vi "Motion_Profile_Setup_Send.vi"(7 "name or relative path":string) -> ()   [LabVIEW 2017]
uses:
  <vilib>/Rock Robotics/WPI/ThirdParty/Phoenix-LabVIEW/Motor Controller/Controls/CTRE_Phoenix_MotorControl_TrajectoryPointTimeDur.ctl
  <vilib>/Utility/file.llb/Read Delimited Spreadsheet (DBL).vi
panel:
  out "Total Run TIme":dbl
  out "Done??":bool
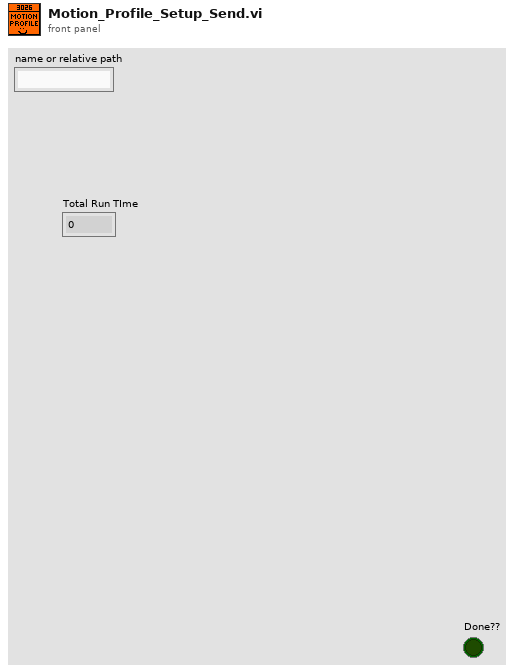
[diagram p1: front panel]
types:
  T1 = typedef "WPI_MotorControlDeviceRef.ctl" = cluster{"DeviceStatus":errorcluster, "Type":T2, "PWM":cluster{"PWM Channel":T3, "DeadBand":T4}, "CAN":cluster{"Device Number":u8, "SetOutput VI Ref":variant, "GetOutput VI Ref":variant, "Enable VI Ref":variant, "Disable VI Ref":variant, "Data":variant}, "Invert":bool, "DIO PWM":cluster{"PWM \"Enable\" Channel":T3, "DIOChannel":T5, "PWM Rate":dbl}}
  T2 = typedef "WPI_MotorControlType.ctl" = enum16{"PWM", "CAN", "DIO PWM"}
  T3 = typedef "FPGA_DIOPWMChannel.ctl" = enum8{"PWM 0", "PWM 1", "PWM 2", "PWM 3", "PWM 4", "PWM 5", "PWM 6", "PWM 7", "PWM 8", "PWM 9", "PWM MXP 0", "PWM MXP 1", "PWM MXP 2", "PWM MXP 3", "PWM MXP 4", "PWM MXP 5", "PWM MXP 6", "PWM MXP 7", "PWM MXP 8", "PWM MXP 9", "Invalid"}
  T4 = typedef "WPI_PWMDeadband.ctl" = cluster{"Name":string, "maxPositivePwm":i32, "minPositivePwm":i32, "centerPwm":i32, "maxNegativePwm":i32, "minNegativePwm":i32, "angularRange":u16}
  T5 = typedef "FPGA_DIOChannel.ctl" = enum8{"DIO 0", "DIO 1", "DIO 2", "DIO 3", "DIO 4", "DIO 5", "DIO 6", "DIO 7", "DIO 8", "DIO 9", "DIO MXP 0", "DIO MXP 1", "DIO MXP 2", "DIO MXP 3", "DIO MXP 4", "DIO MXP 5", "DIO MXP 6", "DIO MXP 7", "DIO MXP 8", "DIO MXP 9", "DIO MXP 10", "DIO MXP 11", "DIO MXP 12", "DIO MXP 13", "DIO MXP 14", "DIO MXP 15", "SPI Port CS1", "SPI Port CS2", "SPI Port CS3", "SPI Port MISO", "SPI Port MOSI", "Invalid"}
  T6 = typedef "CTRE_Phoenix_MotorControl_TrajectoryPointTimeDur.ctl" = i32
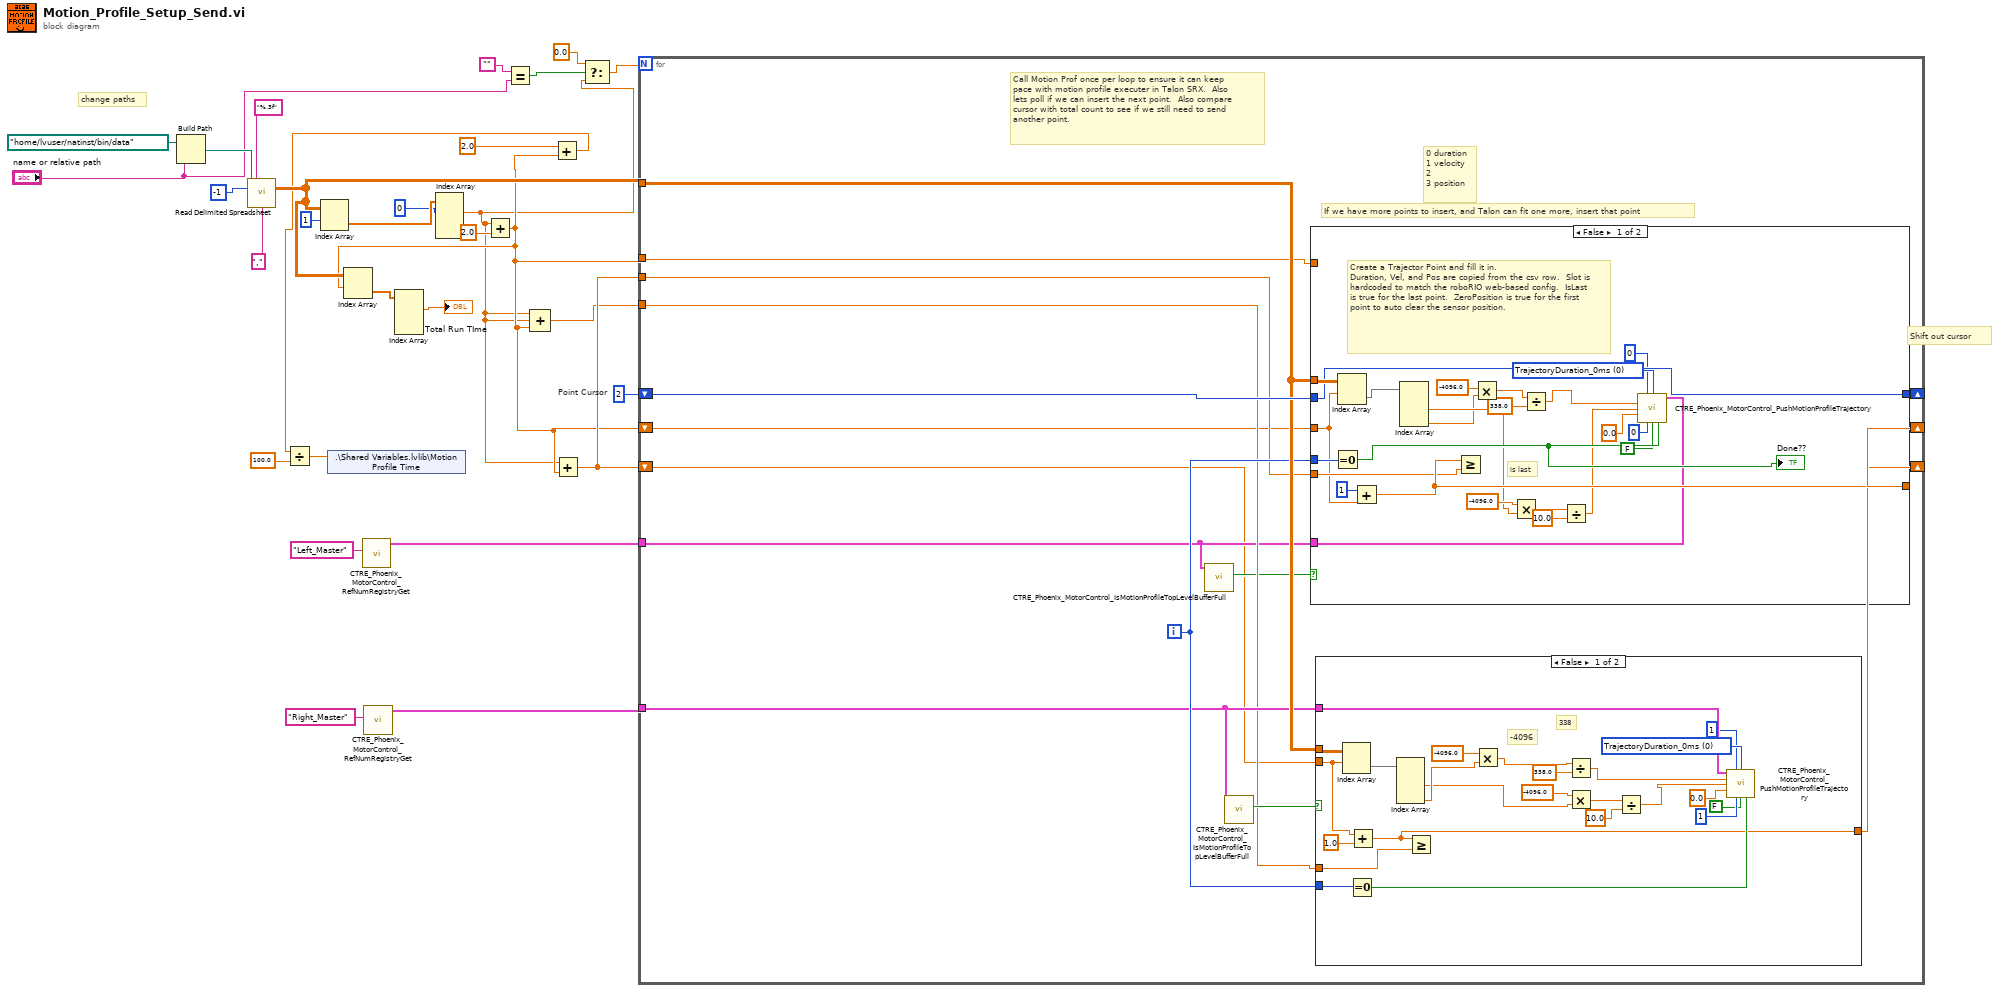
[diagram p0: block diagram]
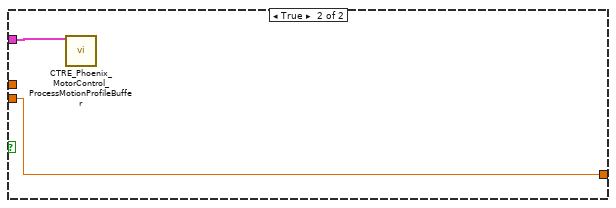
[diagram p2: hidden frame]
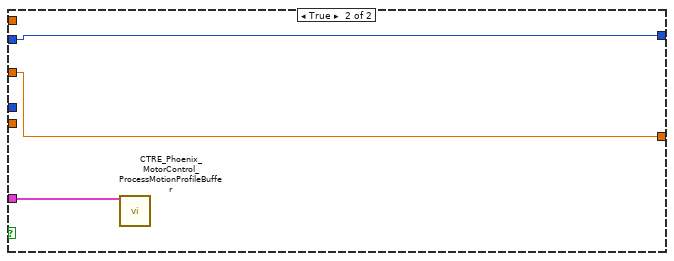
[diagram p3: hidden frame]
diagram:
  w29 = 2  # Point Cursor
  # "change paths"
  # "Shift out cursor"
  n1 = Build Path(base path=path "/home/lvuser/natinst/bin/data", name or relative path="name or relative path") -> (appended path=w28:path)
  n2 = call-poly <vilib>:"Read Delimited Spreadsheet.vi"("file path (dialog if empty)"=w28, "format (%.3f)"="%.3f", "number of rows (all:-1)"=-1, "delimiter (\\t)"="," ("delimiter (\\t)")) -> ("all rows"=w17:dbl[][])  [unwired: 6 in, 5 out]
  n3 = Index Array(array=w17, index (row)=1) -> (element=w25:dbl[])  [unwired: 1 in]
  n4 = call <vilib>:"CTRE_Phoenix_MotorControl_RefNumRegistryGet.vi"("refnum name"="Left_Master") -> ("PhoenixMotorControlDevRef"=w2:T1)  [unwired: 9 in, 1 out]
  n5 = call <vilib>:"CTRE_Phoenix_MotorControl_RefNumRegistryGet.vi"("refnum name"="Right_Master") -> ("PhoenixMotorControlDevRef"=w1:T1)  [unwired: 9 in, 1 out]
  n6 = Index Array(array=w25, index #1=0 ("index")) -> (element #1=w8:dbl)  [unwired: 3 in, 3 out]
  n7 = Add(x=w8, y=2.0) -> (x+y=w15:dbl)
  n8 = Index Array(array=w17, index (row)=w15) -> (element=w16:dbl[])  [unwired: 1 in]
  n9 = Index Array(array=w16) -> (element #1=→"Total Run TIme":dbl)  [unwired: 4 in, 3 out]
  n10 = Equal?(x="", y="name or relative path") -> (x = y?=w4:bool)
  n11 = Compound Arithmetic op=ADD(w8, w8, w15) -> (w18:dbl)
  n12 = Add(x=2.0, y=w15) -> (x+y=w9:dbl)
  n13 = Divide(x=w9, y=100.0) -> (x/y=w11:dbl)
  n14 = shared-variable ".\\Shared Variables.lvlib\\Motion Profile Time"(w11) -> ()  [unwired: 1 in, 1 out]
  n15 = Add(x=w8, y=w15) -> (x+y=w19:dbl)
  n16 = Select(t=0.0, s=w4, f=w8) -> (s? t:f=w7:dbl)
  n17 = for {
    N: w7 -> [_]
    tunnel: w17 -> [w44]
    shift-right: [w33] -> _
    shift-left: w29 -> [w45]
    tunnel: w15 -> [w40]
    tunnel: w2 -> [w37]
    tunnel: w1 -> [w41]
    tunnel: w19 -> [w39]
    tunnel: w18 -> [w38]
    shift-right: [w34] -> _
    shift-left: w19 -> [w31]
    shift-right: [w35] -> _
    shift-left: w15 -> [w32]
    i -> [w43]
    # "0 duration\n1 velocity \n2 \n3 position"
    # "If we have more points to insert, and Talon can fit one more, insert that point"
    # "Call Motion Prof once per loop to ensure it can keep pace with motion profile executer in Talon SRX.  Also lets poll if we can insert the next point.  Also compare cursor with total count to see if we still need to send another point."
    n18 = call <vilib>:"CTRE_Phoenix_MotorControl_IsMotionProfileTopLevelBufferFull.vi"("PhoenixMotorControlDevRef"=w37) -> ("Is Motion Profile Top Level Buffer Full?"=w36:bool)  [unwired: 8 in, 2 out]
    n19 = call <vilib>:"CTRE_Phoenix_MotorControl_IsMotionProfileTopLevelBufferFull.vi"("PhoenixMotorControlDevRef"=w41) -> ("Is Motion Profile Top Level Buffer Full?"=w42:bool)  [unwired: 8 in, 2 out]
    n20 = case shown="False" w36 {
      tunnel: w44 -> [w96 _]
      tunnel: [w93 w99] -> w35
      tunnel: w45 -> [w86 w98]
      tunnel: w37 -> [w87 w97]
      tunnel: w43 -> [w92 _]
      tunnel: w40 -> [_ _]
      tunnel: w39 -> [w88 _]
      tunnel: w32 -> [w75 w99]
      tunnel: [w86 w98] -> w33
      frame False {
        w85 = T6 0 items=["TrajectoryDuration_0ms"=0, "TrajectoryDuration_5ms"=5, "TrajectoryDuration_10ms"=10, "TrajectoryDuration_20ms"=20, "TrajectoryDuration_30ms"=30, "TrajectoryDuration_40ms"=40, "TrajectoryDuration_50ms"=50, "TrajectoryDuration_100ms"=100] ("durationMs")
        # "is last"
        # "Create a Trajector Point and fill it in.\nDuration, Vel, and Pos are copied from the csv row.  Slot is hardcoded to match the roboRIO web-based config.  IsLast is true for the last point.  ZeroPosition is true for the first point to auto clear the sensor position."
        n21 = Equal To 0?(x=w92) -> (x = 0?=w91:bool)
        "Done??" <- w91
        n22 = Index Array(array=w96, index (row)=w75) -> (element=w94:dbl[])  [unwired: 1 in]
        n23 = Add(x=u32 1, y=w75) -> (x+y=w93:dbl)
        n24 = Index Array(array=w94) -> (element #2=w78:dbl, element #4=w77:dbl)  [unwired: 4 in, 2 out]
        n25 = Greater Or Equal?(x=w93, y=w88) -> ()  [unwired: 1 out]
        n26 = Multiply(x=-4096.0, y=w77) -> (x*y=w73:dbl)
        n27 = Multiply(x=-4096.0, y=w78) -> (x*y=w80:dbl)
        n28 = Divide(x=w73, y=338.0) -> (x/y=w72:dbl)
        n29 = Divide(x=w80, y=10.0) -> (x/y=w76:dbl)
        n30 = call <vilib>:"CTRE_Phoenix_MotorControl_PushMotionProfileTrajectory.vi"("PhoenixMotorControlDevRef"=w87, "profileSlotSelect1"=0, "durationMs"=w85, "position"=w72, "velocity"=w76, "headingDeg"=0.0, "profileSlotSelect0"=0 ("profileSlotSelect"), "isLastPoint?"=FALSE, "Zero Position?"=w91) -> ()  [unwired: 5 in, 2 out]
      }
      frame True {
        n31 = call <vilib>:"CTRE_Phoenix_MotorControl_ProcessMotionProfileBuffer.vi"("PhoenixMotorControlDevRef"=w97) -> ()  [unwired: 13 in, 2 out]
      }
    }
    n32 = case shown="False" w42 {
      tunnel: w41 -> [w62 w70]
      tunnel: w44 -> [w69 _]
      tunnel: w43 -> [w67 _]
      tunnel: w38 -> [w61 _]
      tunnel: w31 -> [w49 w71]
      tunnel: [w60 w71] -> w34
      frame False {
        w59 = T6 0 items=["TrajectoryDuration_0ms"=0, "TrajectoryDuration_5ms"=5, "TrajectoryDuration_10ms"=10, "TrajectoryDuration_20ms"=20, "TrajectoryDuration_30ms"=30, "TrajectoryDuration_40ms"=40, "TrajectoryDuration_50ms"=50, "TrajectoryDuration_100ms"=100] ("durationMs")
        # "338"
        # "-4096"
        n33 = Index Array(array=w69, index (row)=w49) -> (element=w68:dbl[])  [unwired: 1 in]
        n34 = Equal To 0?(x=w67) -> (x = 0?=w63:bool)
        n35 = Add(x=w49, y=1.0) -> (x+y=w60:dbl)
        n36 = Index Array(array=w68) -> (element #2=w51:dbl, element #4=w52:dbl)  [unwired: 4 in, 2 out]
        n37 = Greater Or Equal?(x=w60, y=w61) -> ()  [unwired: 1 out]
        n38 = Multiply(x=-4096.0, y=w52) -> (x*y=w48:dbl)
        n39 = Divide(x=w48, y=338.0) -> (x/y=w47:dbl)
        n40 = Multiply(x=-4096.0, y=w51) -> (x*y=w54:dbl)
        n41 = Divide(x=w54, y=10.0) -> (x/y=w50:dbl)
        n42 = call <vilib>:"CTRE_Phoenix_MotorControl_PushMotionProfileTrajectory.vi"("PhoenixMotorControlDevRef"=w62, "profileSlotSelect1"=1, "durationMs"=w59, "position"=w47, "velocity"=w50, "headingDeg"=0.0, "profileSlotSelect0"=1 ("profileSlotSelect"), "isLastPoint?"=FALSE, "Zero Position?"=w63) -> ()  [unwired: 5 in, 2 out]
      }
      frame True {
        n43 = call <vilib>:"CTRE_Phoenix_MotorControl_ProcessMotionProfileBuffer.vi"("PhoenixMotorControlDevRef"=w70) -> ()  [unwired: 13 in, 2 out]
      }
    }
  }
